vi "Method_Const.vi"(4 "Value":dbl, 5 "Input A":refnum<class "Abs_Double Float.lvclass">) -> (1 "Result":T1)   [LabVIEW 2021, in "Subtract_DBL.lvclass"]
uses:
  Subtract_DBL.lvclass
  Abs_Types/Double Float/Abs_Double Float.lvclass
  Abs Type.ctl
  C:/TSA/LV_Abstract/Source/Functions/Support/Function/Two Terminal/DBL/AbsFunc_Two Term_DBL.lvclass
  C:/Program Files (x86)/National Instruments/LabVIEW 2021/vi.lib/TSA/Abstract Data Classes/Abs_Types/Double Float/Abs_Double Float.lvclass
  Support/Function/Two Terminal/DBL/AbsFunc_Two Term_DBL.lvclass/AbsFunc_Two Term_DBL.ctl
  Support/Function/Two Terminal/DBL/Properties/Write Numeric A.vi
  Support/Function/Two Terminal/DBL/Properties/Write Numeric B.vi
  Constants/Support/DBL/Const_DBL.lvclass
  C:/Program Files (x86)/National Instruments/LabVIEW 2021/vi.lib/TSA/Abstract Data Classes/Abs_Types/Numeric/Abs_Numeric.lvclass
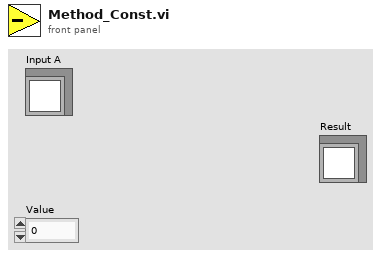
[diagram p1: front panel]
types:
  T1 = typedef "Subtract_DBL.lvclass/Abs Type.ctl" = refnum<class "Abs_Double Float.lvclass">
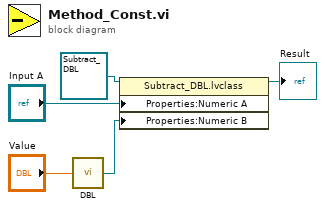
[diagram p0: block diagram]
diagram:
  n1 = call "DBL.vi"("Value"="Value") -> ("Constant"=w2:refnum<class "Const_DBL.lvclass">)  [unwired: 4 in]
  n2 = property class="Subtract_DBL.lvclass"(reference=refnum<class "Subtract_DBL.lvclass"> refnum ("Subtract_DBL.lvclass"), "Properties:Numeric A"="Input A", "Properties:Numeric B"=w2) -> (reference out=→"Result":refnum<class "Subtract_DBL.lvclass">)  [unwired: 1 in, 1 out]
